vi "Get Body Data.vi"(8 "Error In":errorcluster, 11 "Body Reference":refnum<k24>) -> (0 "Error Out":errorcluster, 3 "BodyData":T1)   [LabVIEW 2011, in "LVH-KinectOne.lvlib"]
uses:
  LVH-KinectOne.lvlib
  Type Defs/BodyData.ctl
  Type Defs/ClippedEdges.ctl
  Type Defs/HandLeftConfidence.ctl
  Type Defs/HandLeftState.ctl
  Type Defs/HandRightConfidence.ctl
  Type Defs/HandRightState.ctl
  Microsoft.Kinect
  Type Defs/LeanTrackingState.ctl
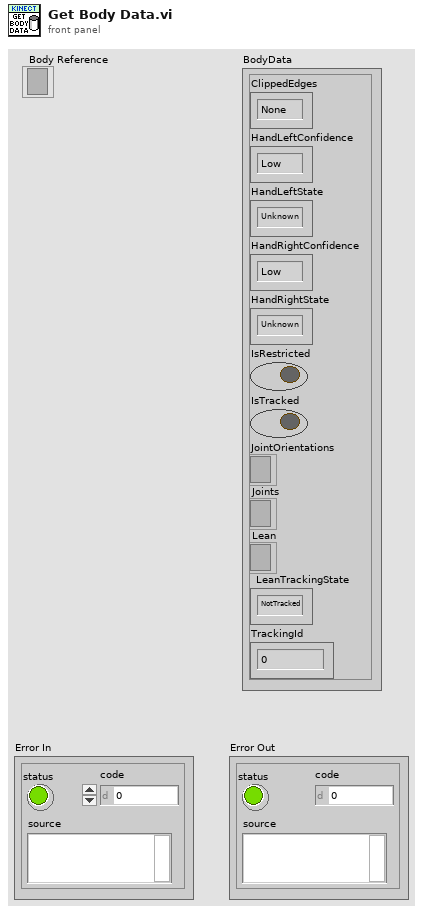
[diagram p1: front panel]
types:
  T1 = typedef "LVH-KinectOne.lvlib/BodyData.ctl" = cluster{"ClippedEdges":T2, "HandLeftConfidence":T3, "HandLeftState":T4, "HandRightConfidence":T5, "HandRightState":T6, "IsRestricted":bool, "IsTracked":bool, "JointOrientations":refnum<k24>, "Joints":refnum<k24>, "Lean":refnum<k24>, "LeanTrackingState":T7, "TrackingId":u64}
  T2 = typedef "LVH-KinectOne.lvlib/ClippedEdges.ctl" = enum16{"None", "Right", "Left", "Top", "Bottom"}
  T3 = typedef "LVH-KinectOne.lvlib/HandLeftConfidence.ctl" = enum16{"Low", "High"}
  T4 = typedef "LVH-KinectOne.lvlib/HandLeftState.ctl" = enum16{"Unknown", "NotTracked", "Open", "Closed", "Lasso"}
  T5 = typedef "LVH-KinectOne.lvlib/HandRightConfidence.ctl" = enum16{"Low", "High"}
  T6 = typedef "LVH-KinectOne.lvlib/HandRightState.ctl" = enum16{"Unknown", "NotTracked", "Open", "Closed", "Lasso"}
  T7 = typedef "LVH-KinectOne.lvlib/LeanTrackingState.ctl" = enum16{"NotTracked", "Inferred", "Tracked"}
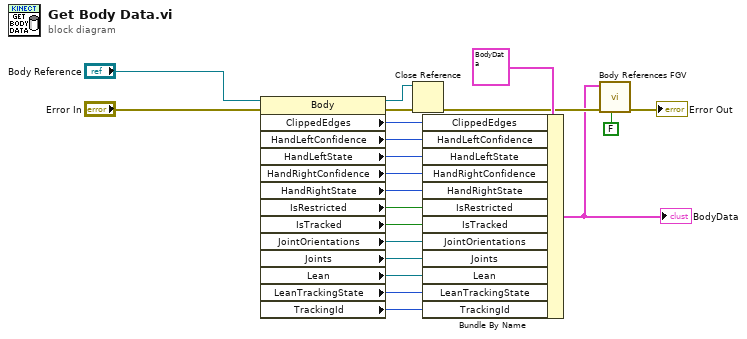
[diagram p0: block diagram]
diagram:
  n1 = property class="Body"(reference="Body Reference", error in="Error In") -> (reference out=w7:refnum<k24>, error out=w8:errorcluster, "ClippedEdges"=w20:i32, "HandLeftConfidence"=w19:i32, "HandLeftState"=w18:i32, "HandRightConfidence"=w17:i32, "HandRightState"=w16:i32, "IsRestricted"=w15:bool, "IsTracked"=w14:bool, "JointOrientations"=w13:refnum<k24>, "Joints"=w12:refnum<k24>, "Lean"=w11:refnum<k24>, "LeanTrackingState"=w10:i32, "TrackingId"=w9:u64)
  n2 = Close Reference(reference=w7, error in (no error)=w8) -> (error out=w5:errorcluster)
  n3 = Bundle By Name(cluster=T1 {"ClippedEdges"=enum."None", "HandLeftConfidence"=enum."Low", "HandLeftState"=enum."Unknown", "HandRightConfidence"=enum."Low", "HandRightState"=enum."Unknown", "IsRestricted"=FALSE, "IsTracked"=FALSE, "JointOrientations"=refnum, "Joints"=refnum, "Lean"=refnum, "LeanTrackingState"=enum."NotTracked", "TrackingId"=0} ("BodyData"), "ClippedEdges"=w20, "HandLeftConfidence"=w19, "HandLeftState"=w18, "HandRightConfidence"=w17, "HandRightState"=w16, "IsRestricted"=w15, "IsTracked"=w14, "JointOrientations"=w13, "Joints"=w12, "Lean"=w11, "LeanTrackingState"=w10, "TrackingId"=w9) -> (w3:T1)
  "BodyData" <- w3
  n4 = call "Body References FGV.vi"("Destroy References?"=FALSE, "error in (no error)"=w5, "BodyData"=w3) -> ("error out"=→"Error Out":errorcluster)  [unwired: 8 in]
